vi "Wave2D_Cal QU.vi"(10 "Q":T2, 11 "U":dbl[][](array[numeric])) -> (0 "error":i32, 3 "QU":dbl[][](array[numeric]))   [LabVIEW 2020, in "NI_PDE.lvlib"]
uses:
  <vilib>/gmath/NI_PDE.lvlib
  <vilib>/Analysis/Matrix/Datatypes/RealMatrix.ctl
  <vilib>/Analysis/baseanly.llb/Real A x B.vi
  <vilib>/Analysis/NI_AALBase.lvlib
  <vilib>/Analysis/Matrix/NI_Matrix.lvlib
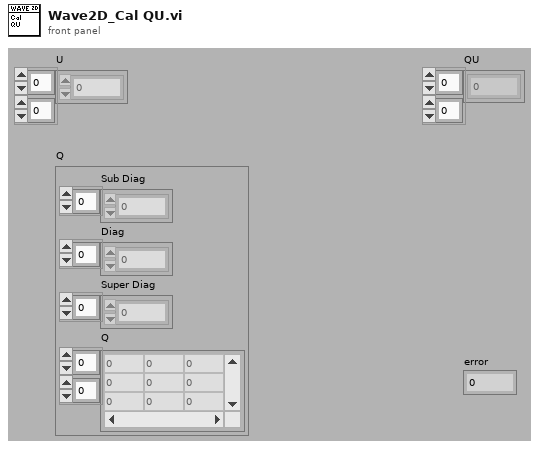
[diagram p1: front panel]
types:
  T1 = typedef "NI_Matrix.lvlib/RealMatrix.ctl" = dbl[][]
  T2 = cluster{"Sub Diag":dbl[], "Diag":dbl[], "Super Diag":dbl[], "Q":T1}
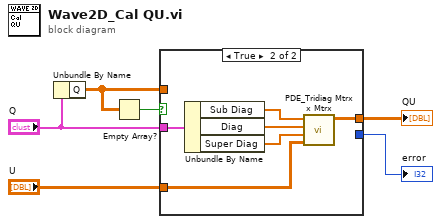
[diagram p0: block diagram]
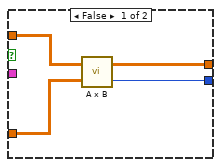
[diagram p2: hidden frame]
diagram:
  n1 = Unbundle By Name("Q") -> ("Q"=w4:T1)
  n2 = Empty Array?(array=w4) -> (empty?=w6:bool)
  n3 = case shown="True" w6 {
    tunnel: "U" -> [w9 w12]
    tunnel: w4 -> [w10 _]
    tunnel: [w8 w11] -> w3
    tunnel: [w7 _] -> w1
    tunnel: "Q" -> [_ w16]
    frame False {
      n4 = call-poly <vilib>:"A x B.vi"("B"=w9, "A"=w10) -> ("error"=w7:i32, "A x B"=w8:T1)
    }
    frame True {
      n5 = Unbundle By Name(w16) -> ("Sub Diag"=w15:dbl[], "Diag"=w14:dbl[], "Super Diag"=w13:dbl[])
      n6 = call <vilib>:"PDE_Tridiag Mtrx x Mtrx.vi"("X"=w12, "Super Diag"=w13, "Diag"=w14, "Sub Diag"=w15) -> ("Mtrx x X"=w11:dbl[][])  [unwired: 7 out]
    }
  }
  "QU" <- w3
  "error" <- w1
